vi "Color to bool array.vi"(8 "error in (no error)":errorcluster, 11 "Calib color":T1) -> (0 "error out":errorcluster, 3 "LED Panel 2":T2)   [LabVIEW 2020]
uses:
  Controls/LED panel ---typedef.ctl
  Controls/Calibration color ---typedef.ctl
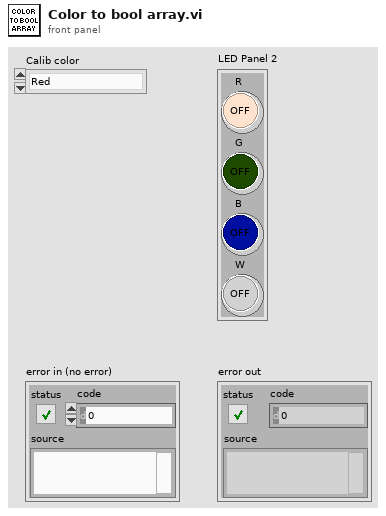
[diagram p1: front panel]
types:
  T1 = typedef "Calibration color ---typedef.ctl" = enum16{"Red", "Green", "Blue", "White"}
  T2 = typedef "LED panel ---typedef.ctl" = cluster{"R":bool, "G":bool, "B":bool, "W":bool}
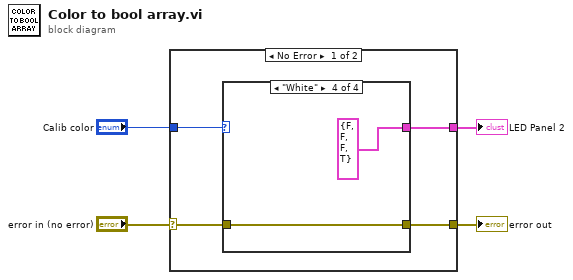
[diagram p0: block diagram]
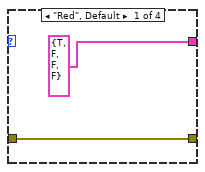
[diagram p2: hidden frame]
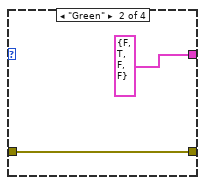
[diagram p3: hidden frame]
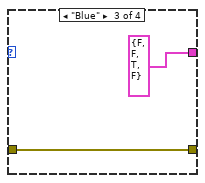
[diagram p4: hidden frame]
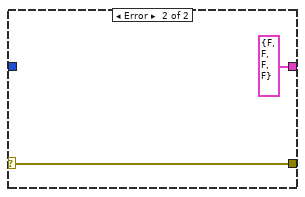
[diagram p5: hidden frame]
diagram:
  n1 = case shown="No Error" "error in (no error)" {
    selector: "error in (no error)" -> [w6 w18]
    tunnel: "Calib color" -> [w8 _]
    tunnel: [w7 T2 {"R"=FALSE, "G"=FALSE, "B"=FALSE, "W"=FALSE} ("LED Panel 3")] -> w3
    tunnel: [w5 w18] -> w1
    frame No Error {
      n2 = case shown="\"White\"" w8 {
        tunnel: [T2 {"R"=TRUE, "G"=FALSE, "B"=FALSE, "W"=FALSE} ("LED Panel 3") T2 {"R"=FALSE, "G"=TRUE, "B"=FALSE, "W"=FALSE} ("LED Panel 3") T2 {"R"=FALSE, "G"=FALSE, "B"=TRUE, "W"=FALSE} ("LED Panel 3") T2 {"R"=FALSE, "G"=FALSE, "B"=FALSE, "W"=TRUE} ("LED Panel 3")] -> w7
        tunnel: w6 -> [w9 w11 w13 w15]
        tunnel: [w9 w11 w13 w15] -> w5
        frame "Red", Default {
        }
        frame "Green" {
        }
        frame "Blue" {
        }
        frame "White" {
        }
      }
    }
    frame Error {
    }
  }
  "LED Panel 2" <- w3
  "error out" <- w1
